vi "UpdateAttribute.vi"(8 "error in (no error)":errorcluster, 9 "Attribute Name":string, 10 "Attribute":refnum<class "Attribute.lvclass">, 11 "SMO in":refnum<class "SMO.lvclass">) -> (0 "error out":errorcluster, 2 "replaced":bool, 3 "SMO out":refnum<class "SMO.lvclass">)   [LabVIEW 2021, in "smo.lvlib" / "SMO.lvclass"]
uses:
  SMO.lvclass
  Support/Attribute/Attribute.lvclass
  SMO.lvclass/SMO.ctl
  Support/Attribute/Attribute.lvclass/Attribute.ctl
  <vilib>/Utility/LVClass/Get LV Class Name.vi
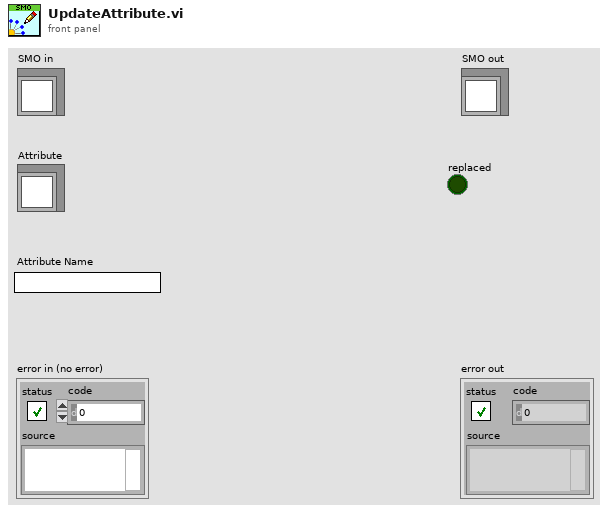
[diagram p1: front panel]
types:
  T1 = typedef "smo.lvlib/SMO.lvclass/PrivateData--Ref.ctl" = refnum<data-value>
  T2 = typedef "smo.lvlib/SMO.lvclass/PrivateData--Cluster.ctl" = cluster{"Parent Call":T3, "Registered Processes":T4[], "Sync Notifier":refnum<notifier>, "Process Error Notifier":refnum<notifier>, "Protected Events":T5, "Public Events":T6, "SMO State":T7, "[Attributes]":variant, "Launcher Close":refnum<notifier>, "Caller Watchdog":refnum<queue>, "Accessibility":T8, "NbStaticDependencies":u32}
  T3 = typedef "smo.lvlib/SMO.lvclass/Parent Call--Enum.ctl" = enum16{"Allows parent to run", "Does not request parent to run"}
  T4 = typedef "smo.lvlib/SMO.lvclass/RegisteredProcessData--Cluster.ctl" = cluster{"Name":string, "Static VI Ref":refnum<vi>, "Running":bool, "NotifierRef":u32}
  T5 = typedef "smo.lvlib/SMO.lvclass/Protected Events.ctl" = cluster{"StopProcesses":refnum<user-event>, "AbortProcesses":refnum<user-event>, "Config Changed":refnum<user-event>, "Dependency":refnum<user-event>}
  T6 = typedef "smo.lvlib/SMO.lvclass/Public Events.ctl" = cluster{"Error":refnum<user-event>, "State":refnum<user-event>, "Reserve State":refnum<user-event>}
  T7 = typedef "smo.lvlib/SMO.lvclass/SMOState --Enum.ctl" = enum16{"unknown", "Created", "Started", "Stopped"}
  T8 = typedef "smo.lvlib/SMO.lvclass/Accessibility--Cluster.ctl" = cluster{"Lock Key":string, "Reserve State":T9}
  T9 = typedef "smo.lvlib/SMO.lvclass/Reserve State--Enum.ctl" = enum16{"Unreserved", "Reserved", "Self-locked"}
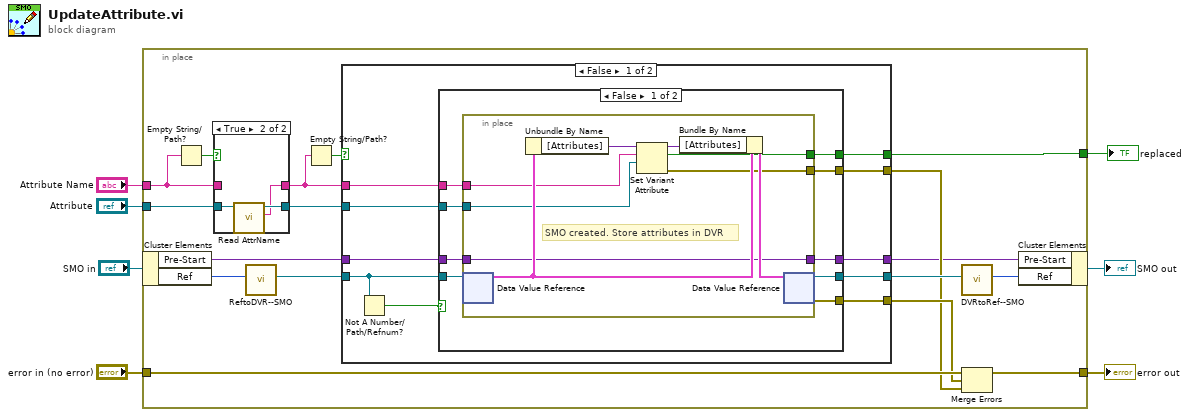
[diagram p0: block diagram]
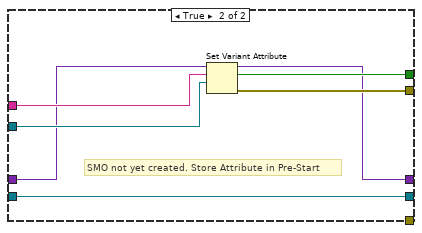
[diagram p2: hidden frame]
diagram:
  n1 = in-place {
    in-place-border: "error in (no error)" -> [w20]
    in-place-border: [w18] -> w4
    in-place-border: "Attribute" -> [w14]
    in-place-border: "Attribute Name" -> [w15]
    in-place-border: [w10] -> w1
    n2 = in-place-cluster #1("SMO in") -> ("Pre-Start"=w9:variant, "Ref"=w24:u32)
    n3 = Empty String/Path?(string/path=w15) -> (empty?=w16:bool)
    n4 = case shown="True" w16 {
      tunnel: w15 -> [w63 _]
      tunnel: [w63 w64] -> w12
      tunnel: w14 -> [w62 w66]
      tunnel: [w62 w65] -> w13
      frame False {
      }
      frame True {
        n5 = call "Read AttrName.vi"("Attribute in"=w66) -> ("Attribute Name"=w64:string, "Attribute out"=w65:refnum<class "Attribute.lvclass">)  [unwired: 8 in, 1 out]
      }
    }
    n6 = call "ReftoDVR--SMO.vi"("Ref"=w24) -> ("Ref"=w23:T1)  [unwired: 10 in]
    n7 = Empty String/Path?(string/path=w12) -> (empty?=w11:bool)
    n8 = case shown="False" w11 {
      tunnel: w23 -> [w28 w61]
      tunnel: [w34 w61] -> w22
      tunnel: [w33 _] -> w19
      tunnel: [w32 _] -> w17
      tunnel: w13 -> [w31 _]
      tunnel: w12 -> [w30 _]
      tunnel: [w29 _] -> w10
      tunnel: w9 -> [w26 w60]
      tunnel: [w25 w60] -> w8
      frame False {
        n9 = Not A Number/Path/Refnum?(number/path/refnum=w28) -> (NaN/Path/Refnum?=w27:bool)
        n10 = case shown="False" w27 {
          tunnel: [w43 w53] -> w34
          tunnel: [w42 _] -> w33
          tunnel: [w41 w59] -> w32
          tunnel: w31 -> [w40 w58]
          tunnel: w30 -> [w39 w57]
          tunnel: [w38 w56] -> w29
          tunnel: w28 -> [w37 w53]
          tunnel: w26 -> [w36 w55]
          tunnel: [w35 w54] -> w25
          frame False {
            n11 = in-place {
              in-place-border: w40 -> [w47]
              in-place-border: w39 -> [w48]
              in-place-border: [w46] -> w41
              in-place-border: [w45] -> w38
              in-place-border: w36 -> [w44]
              in-place-border: [w44] -> w35
              # "SMO created. Store attributes in DVR"
              n12 = in-place-dvr #2(w37) -> (w51:T2)  [unwired: 1 out]
              n13 = Unbundle By Name(w51) -> ("[Attributes]"=w50:variant)
              n14 = Set Variant Attribute(Variant=w50, name=w48, value=w47) -> (Variant out=w49:variant, replaced=w45:bool, error out=w46:errorcluster)  [unwired: 1 in]
              n15 = Bundle By Name(cluster=w51, "[Attributes]"=w49) -> (w52:T2)
              n16 = in-place-dvr #2(w52) -> (w43:T1, w42:errorcluster)
            }
          }
          frame True {
            # "SMO not yet created. Store Attribute in Pre-Start"
            n17 = Set Variant Attribute(Variant=w55, name=w57, value=w58) -> (Variant out=w54:variant, replaced=w56:bool, error out=w59:errorcluster)  [unwired: 1 in]
          }
        }
      }
      frame True {
      }
    }
    n18 = call "DVRtoRef--SMO.vi"("Ref"=w22) -> ("Ref"=w21:u32)  [unwired: 10 in]
    n19 = Merge Errors(w20, w19, w17) -> (w18:errorcluster)
    n20 = in-place-cluster #1("Pre-Start"=w8, "Ref"=w21) -> (→"SMO out":refnum<class "SMO.lvclass">)
  }
  "error out" <- w4
  "replaced" <- w1
